vi "Write url 1.vi"(8 "error in (no error)":errorcluster, 10 "url":string, 11 "Firebase in":refnum<class "Firebase.lvclass">) -> (0 "error out":errorcluster, 3 "Firebase out":refnum<class "Firebase.lvclass">)   [LabVIEW 2019, in "Firebase.lvclass"]
uses:
  Firebase.lvclass
  Firebase.lvclass/Firebase.ctl
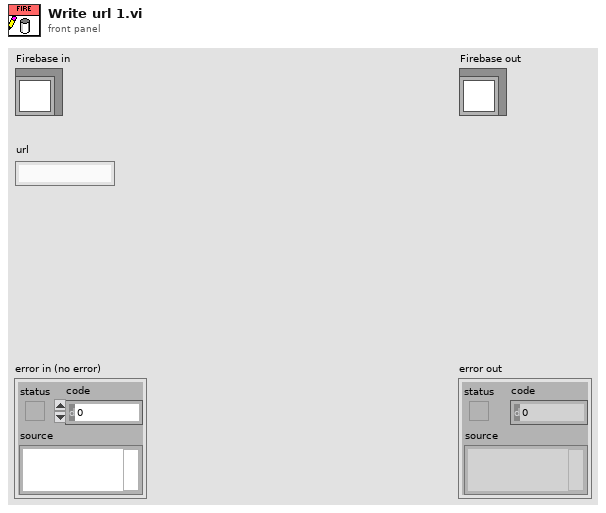
[diagram p1: front panel]
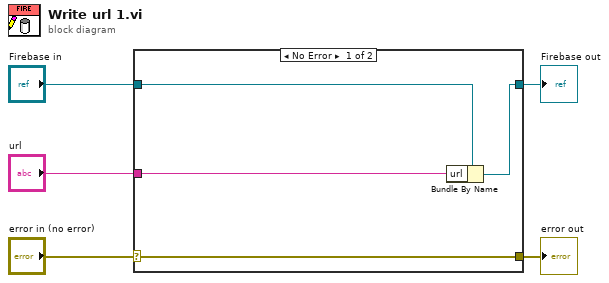
[diagram p0: block diagram]
diagram:
  n1 = case shown="No Error" "error in (no error)" {
    selector: "error in (no error)" -> [w9 w10]
    tunnel: [w9 w10] -> w4
    tunnel: [w7 w11] -> w2
    tunnel: "Firebase in" -> [w8 w11]
    tunnel: "url" -> [w6 _]
    frame No Error {
      n2 = Bundle By Name(cluster=w8, "url"=w6) -> (w7:refnum<class "Firebase.lvclass">)
    }
    frame Error {
    }
  }
  "error out" <- w4
  "Firebase out" <- w2
